vi "NI 9411_READ.vi"(0 "Refnum in":refnum<k21>, 1 "lower limit":dbl, 5 "upper limit":dbl, 11 "Array In":dbl[](array[numeric]), 12 "frequency Feedback":dbl, 13 "error in (no error)":errorcluster) -> (3 "task out":refnum<k21>, 4 "RPM":dbl, 6 "Media":dbl, 10 "frequency":dbl, 14 "error out":errorcluster, 15 "Array out":dbl[](array[numeric]))   [LabVIEW 2019]
uses:
  <vilib>/DAQmx/read.llb/DAQmx Read (Counter DBL 1Chan 1Samp).vi
  <vilib>/DAQmx/miscellaneous.llb/DAQmx Fill In Error Info.vi
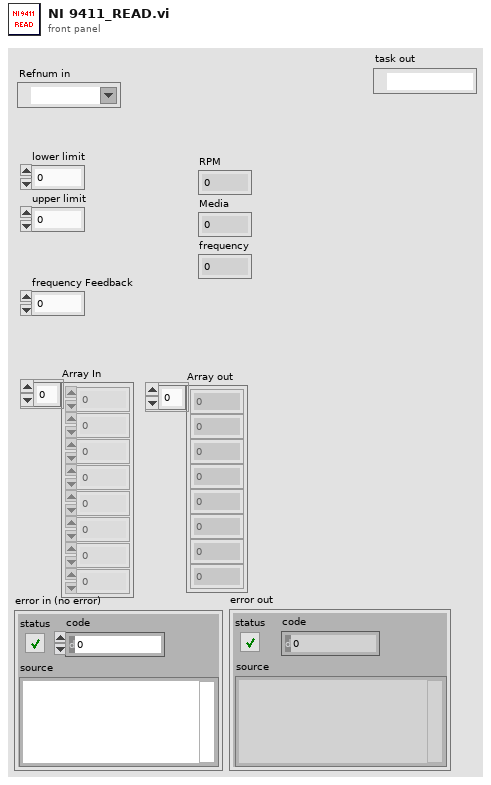
[diagram p1: front panel]
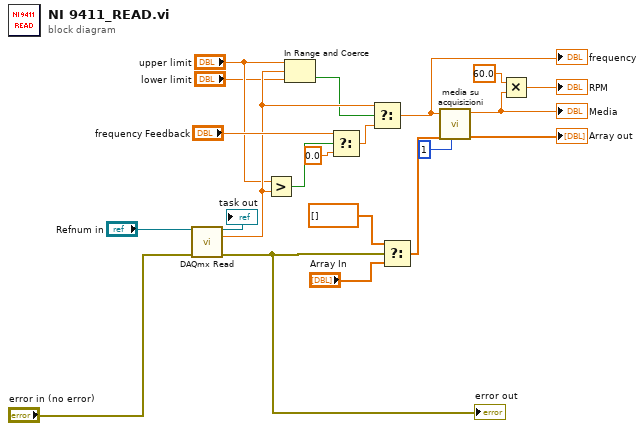
[diagram p0: block diagram]
diagram:
  n1 = call-poly <vilib>:"DAQmx Read.vi"("task/channels in"="Refnum in", "error in"="error in (no error)") -> ("task out"=→"task out":refnum<k21>, "data"=w12:dbl, "error out"=w2:errorcluster)  [unwired: 11 in]
  "error out" <- w2
  n2 = Greater?(x="upper limit", y=w12) -> (0:w13:bool)
  n3 = In Range and Coerce(upper limit="upper limit", x=w12, lower limit="lower limit") -> (In Range?=w10:bool)  [unwired: 1 out]
  n4 = Select(t="frequency Feedback", s=w13, f=0.0) -> (s? t:f=w16:dbl)
  n5 = Select(t=w12, s=w10, f=w16) -> (s? t:f=w17:dbl)
  "frequency" <- w17
  n6 = Select(t=dbl[] [], s=w2, f="Array In") -> (s? t:f=w5:dbl[])
  n7 = call <userlib>:"media su acquisizioni.vi"("n°campioni"=1, "Array ing"=w5, "Value"=w17) -> ("Array out"=→"Array out":dbl[], "Media"=w18:dbl)  [unwired: 5 in, 2 out]
  "Media" <- w18
  n8 = Multiply(x=60.0, y=w18) -> (x*y=→"RPM":dbl)
